vi "Dodanie zaznaczonego punktu na podstawie odległości.vi"(6 "output array in":string[][](array[string]), 8 "Pocz. poł.":T1 {"UTM"."N [m]" format="%#_10g"}, 9 "Obsługa punktów":T2, 10 "Parametry odwzorowania Ziemi (WGS84)":cluster{"a":dbl, "b":dbl}, 11 "Ring in":refnum<vi>) -> (4 "output array out":string[][](array[string]))   [LabVIEW 2012, in "Biblioteka moduł map v3.lvlib" / "Pomocnicze.lvlib"]
doc: "Dodaje do listy współrzędnych ostatnio zaznaczony punkt na mapie. Wyznacza odległość względem punktu startowego z wykorzystaniem odległości przy"
uses:
  Pomocnicze.lvlib
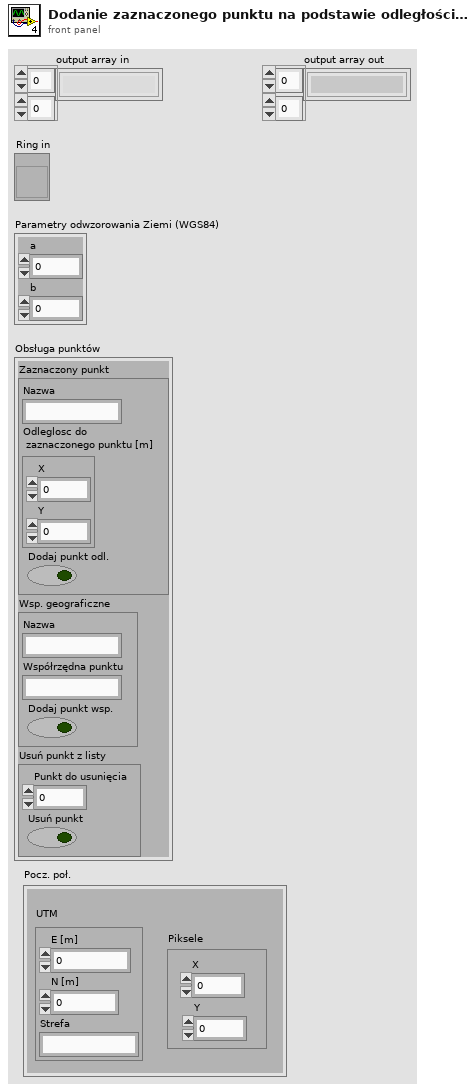
[diagram p1: front panel]
types:
  T1 = cluster{"UTM":cluster{"E [m]":ext, "N [m]":ext, "Strefa":string}, "Piksele":cluster{"X":i32, "Y":i32}}
  T2 = cluster{"Zaznaczony punkt":cluster{"Nazwa":string, "Odleglosc do\n zaznaczonego punktu [m]":cluster{"X":dbl, "Y":dbl}, "Dodaj punkt odl.":bool}, "Wsp. geograficzne":cluster{"Nazwa":string, "Współrzędna punktu":string, "Dodaj punkt wsp.":bool}, "Usuń punkt z listy":cluster{"Punkt do usunięcia":u16, "Usuń punkt":bool}}
  T3 = cluster{"Nazwa zaznaczonego punktu":string, "Odleglosc do\n zaznaczonego punktu [m]":cluster{"X":dbl, "Y":dbl}}
  T4 = cluster{"E [m]":ext, "N [m]":ext, "Strefa":string}
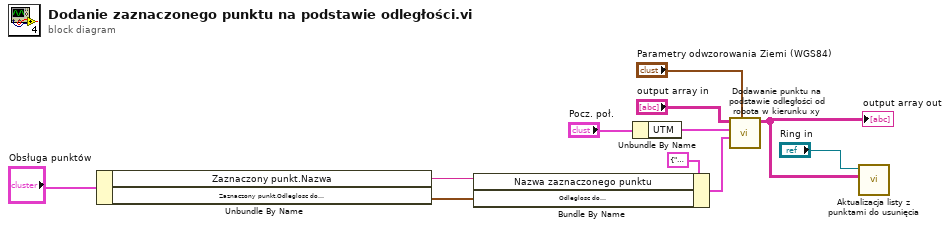
[diagram p0: block diagram]
diagram:
  n1 = Unbundle By Name("Obsługa punktów") -> ("Zaznaczony punkt.Nazwa"=w10:string, "Zaznaczony punkt.Odleglosc do\n zaznaczonego punktu [m]"=w11:cluster{"X":dbl, "Y":dbl})
  n2 = Bundle By Name(cluster=T3 {"Nazwa zaznaczonego punktu"="er", "Odleglosc do\n zaznaczonego punktu [m]"={"X"=23.89186471933565, "Y"=43.80175198544869}} ("Zaznaczony punkt"), "Nazwa zaznaczonego punktu"=w10, "Odleglosc do\n zaznaczonego punktu [m]"=w11) -> (w4:T3)
  n3 = Unbundle By Name("Pocz. poł.") -> ("UTM"=w8:T4)
  n4 = call "Dodawanie punktu na podstawie odległości od robota w kierunku xy.vi"("Parametry odwzorowania Ziemi"="Parametry odwzorowania Ziemi (WGS84)", "Zaznaczony punkt"=w4, "Początkowe UTM"=w8, "Lista współrzędnych"="output array in") -> ("output array"=w7:string[][])  [unwired: 7 in]
  "output array out" <- w7
  n5 = call "Aktualizacja listy z punktami do usunięcia.vi"("Lista współrzędnych"=w7, "Lista z punktami do usunięcia"="Ring in") -> ()  [unwired: 10 in]
